vi "Add Project Item.vi"(8 "error in (no error)":errorcluster, 10 "Folder Location Ref":refnum<vi>, 11 "EST Output in":refnum<class "EST Output.lvclass">) -> (0 "error out":errorcluster, 3 "EST Output out":refnum<class "EST Output.lvclass">)   [LabVIEW 2015, in "EST Output.lvclass"]
uses:
  EST Output.lvclass
  EST Output.lvclass/EST Output.ctl
  IO Class/Read Signal Name.vi
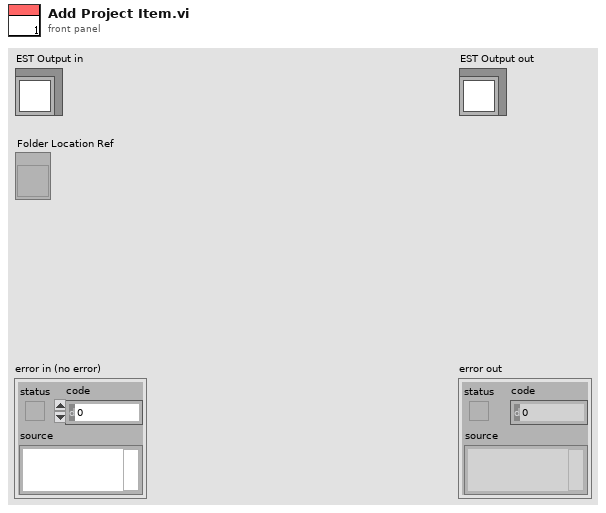
[diagram p1: front panel]
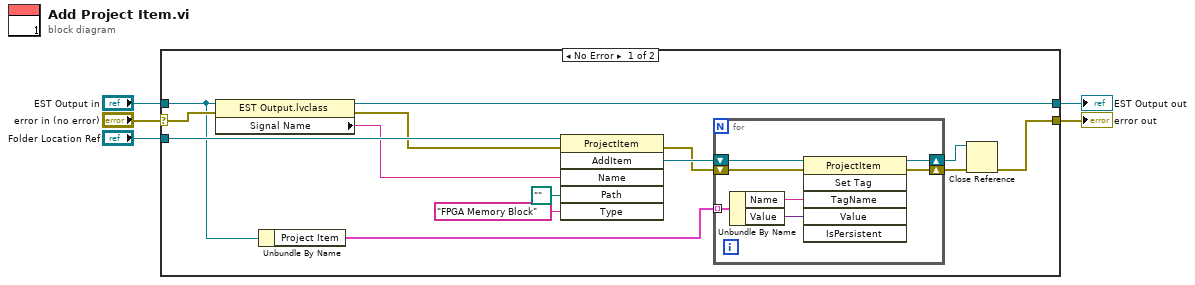
[diagram p0: block diagram]
diagram:
  n1 = case shown="No Error" "error in (no error)" {
    selector: "error in (no error)" -> [w10 w28]
    tunnel: [w12 w28] -> w3
    tunnel: "Folder Location Ref" -> [w13 _]
    tunnel: "EST Output in" -> [w8 w27]
    tunnel: [w6 w27] -> w4
    frame No Error {
      n2 = property class="EST Output.lvclass"(reference=w8, error in=w10) -> (reference out=w6:refnum<class "EST Output.lvclass">, error out=w9:errorcluster, "Signal Name"=w11:string)
      n3 = Unbundle By Name(w8) -> ("Project Item"=w7:cluster{"Name":string, "Value":variant}[])
      n4 = invoke class="ProjectItem" method="AddItem"(reference=w13, error in=w9, "Name"=w11, "Path"=path "", "Type"="FPGA Memory Block") -> (error out=w16:errorcluster, "AddItem"=w18:refnum<vi>)  [unwired: 1 in, 4 out]
      n5 = for {
        shift-right: [w21] -> w14
        shift-left: w16 -> [w25]
        tunnel: w7 -> [w24] mode=indexing
        shift-right: [w20] -> w15
        shift-left: w18 -> [w26]
        n6 = Unbundle By Name(w24) -> ("Name"=w23:string, "Value"=w22:variant)
        n7 = invoke class="ProjectItem" method="Set Tag"(reference=w26, error in=w25, "TagName"=w23, "Value"=w22) -> (reference out=w20:refnum<vi>, error out=w21:errorcluster)  [unwired: 2 in, 4 out]
      }
      n8 = Close Reference(reference=w15, error in (no error)=w14) -> (error out=w12:errorcluster)
    }
    frame Error {
    }
  }
  "error out" <- w3
  "EST Output out" <- w4
